vi "Diagnostic Sample.vi"(8 "error in (no error)":errorcluster, 10 "Acquisition Data in":T1, 11 "DriverMasterSync in":refnum<class "DriverMasterSync.lvclass">) -> (0 "error out":errorcluster, 2 "Acquisition Data out":T1, 3 "DriverMasterSync out":refnum<class "DriverMasterSync.lvclass">)   [LabVIEW 2014, in "DriverMasterSync.lvlib" / "DriverMasterSync.lvclass"]
uses:
  DriverMasterSync.lvclass
  APIs/Data Queue/Acquisition Data Cluster.ctl
  APIs/Data Queue/Acquisition Data 1 Sample Cluster.ctl
  APIs/Data Queue/WINFAS 2 Data Queue.lvlib
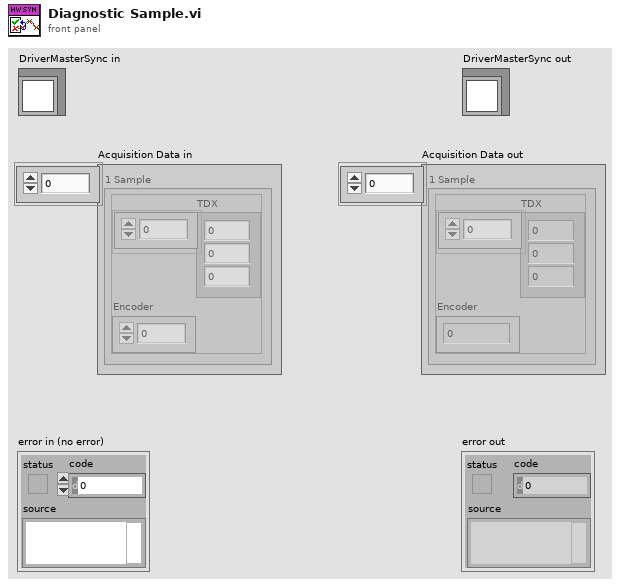
[diagram p1: front panel]
types:
  T1 = typedef "WINFAS 2 Data Queue.lvlib/Acquisition Data Cluster.ctl" = T2[]
  T2 = typedef "WINFAS 2 Data Queue.lvlib/Acquisition Data 1 Sample Cluster.ctl" = cluster{"TDX":sgl[], "Encoder":sgl}
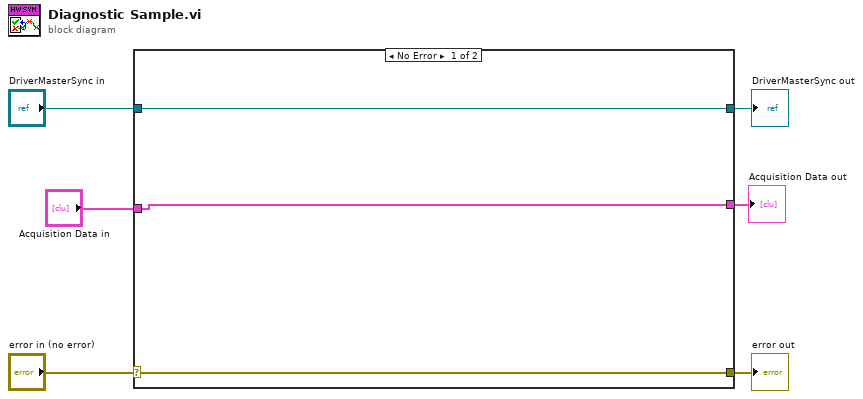
[diagram p0: block diagram]
diagram:
  n1 = case shown="No Error" "error in (no error)" {
    selector: "error in (no error)" -> [w8 w11]
    tunnel: [w8 w11] -> w5
    tunnel: [w9 w10] -> w3
    tunnel: "DriverMasterSync in" -> [w9 w10]
    tunnel: "Acquisition Data in" -> [w7 _]
    tunnel: [w7 _] -> w1
    frame No Error {
    }
    frame Error {
    }
  }
  "error out" <- w5
  "DriverMasterSync out" <- w3
  "Acquisition Data out" <- w1
